vi "enable&disable calibration control by step.vi"(10 "Step Number":i32, 11 "Reference array":refnum<vi>[](array[refnum])) -> ()   [LabVIEW 2020]
doc: "Этот подприбор обеспечивает блокировку/разблокировку контролов окна калибровки. Ссылки на контролы (по 2 на каждый шаг) упорядоченно собраны в массив на vi графического интерфеса. Для выбранного шага контролы разблокируются, остальные контролы блокируются"
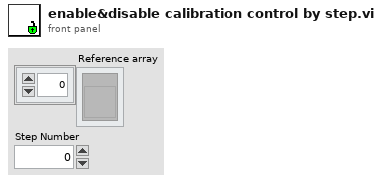
[diagram p1: front panel]
types:
  T1 = enum8{"Enabled", "Disabled", "Disabled and Grayed Out"}
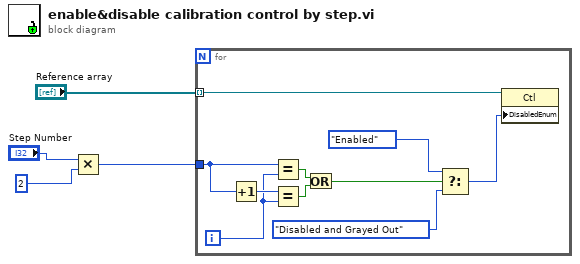
[diagram p0: block diagram]
diagram:
  n1 = Multiply(x="Step Number", y=2) -> (x*y=w1:i32)
  n2 = for {
    tunnel: "Reference array" -> [w5] mode=indexing
    tunnel: w1 -> [w13]
    i -> [w12]
    n3 = Increment(x=w13) -> (x+1=w14:i32)
    n4 = Equal?(x=w13, y=w12) -> (x = y?=w11:bool)
    n5 = Equal?(x=w14, y=w12) -> (x = y?=w10:bool)
    n6 = Or(x=w11, y=w10) -> (x .or. y?=w9:bool)
    n7 = Select(t=T1."Enabled" ("Disabled"), s=w9, f=T1."Disabled and Grayed Out" ("Disabled")) -> (s? t:f=w6:T1)
    n8 = property class="Ctl"(reference=w5, "DisabledEnum"=w6) -> ()  [unwired: 1 in, 2 out]
  }
